vi "LockinDAQ.Trigger.vi"(8 "error in (no error)":errorcluster, 11 "LockinDAQ":refnum<class "LockinDAQ.lvclass">) -> (0 "error out":errorcluster, 3 "LockinDAQ out":refnum<class "LockinDAQ.lvclass">)   [LabVIEW 2016, in "LockinDAQ.lvclass"]
uses:
  LockinDAQ.lvclass
  Typedefs/DAQType-enum.ctl
  LockinDAQ.lvclass/LockinDAQ.ctl
  <vilib>/DAQmx/configure/trigger.llb/DAQmx Start Trigger (Digital Edge).vi
  <resource>/objmgr/daqmx.rc
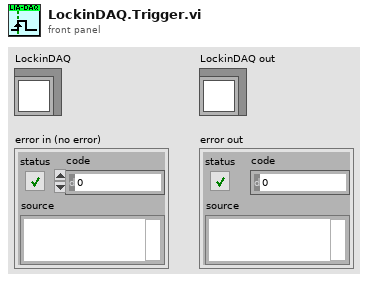
[diagram p1: front panel]
types:
  T1 = typedef "LockinDAQ.lvclass/DAQType-enum.ctl" = enum16{"None", "USB 4431", "PXI 446x"}
  T2 = cluster{"DAQ Type":T1, "master task":refnum<k21>, "RefClk.Src":tag, "SyncPulse.Src":tag, "Trigger.Src":tag, "SyncPulse.SyncTime":dbl}
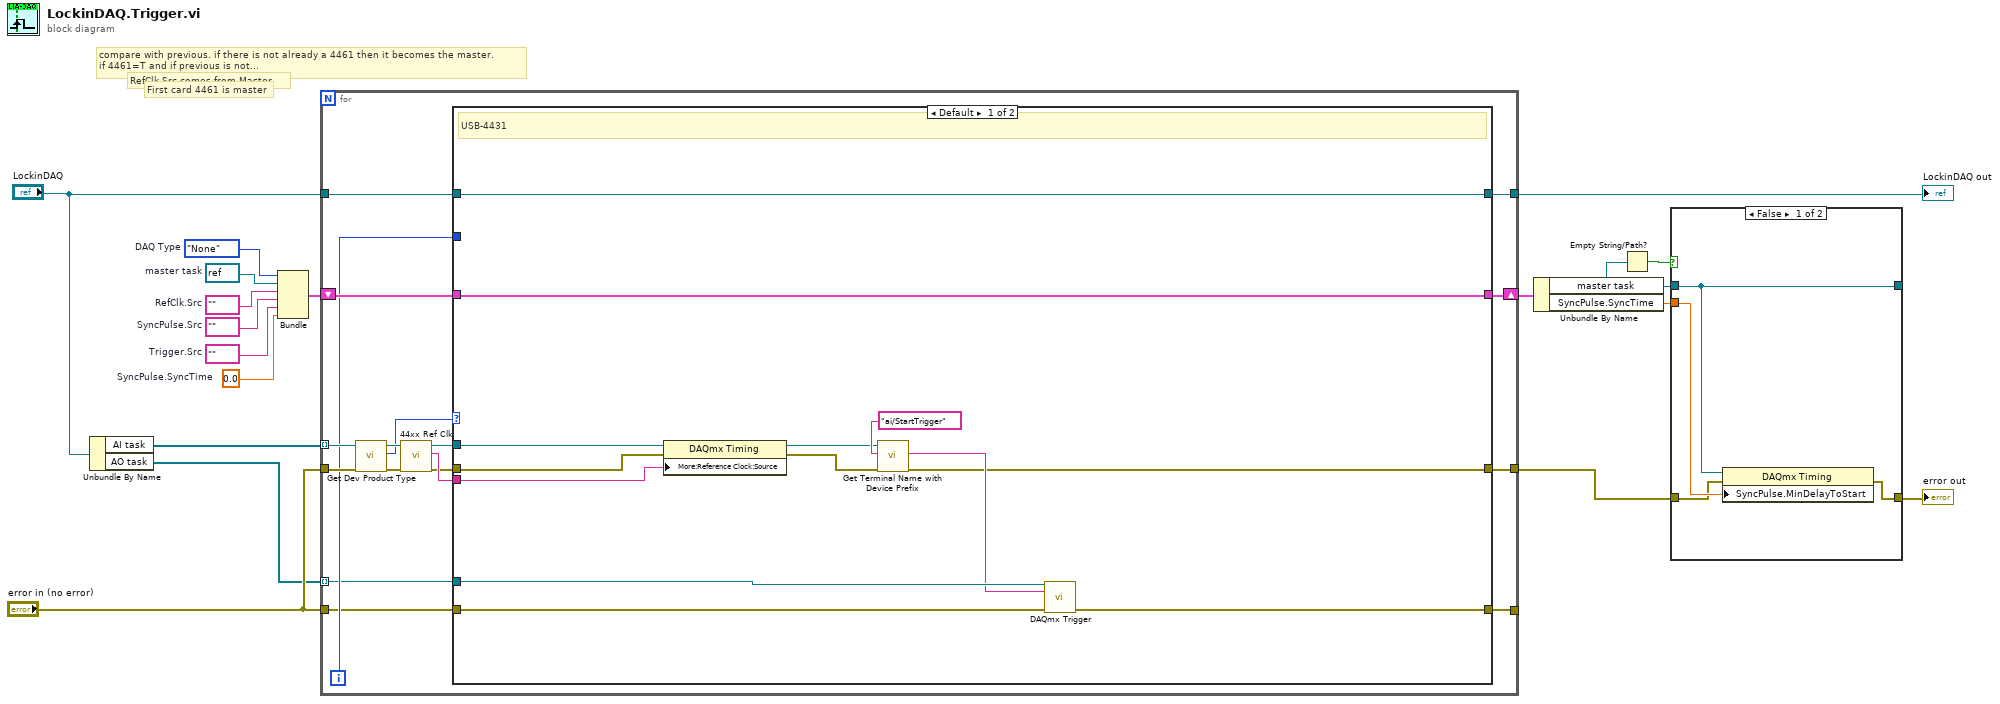
[diagram p0: block diagram]
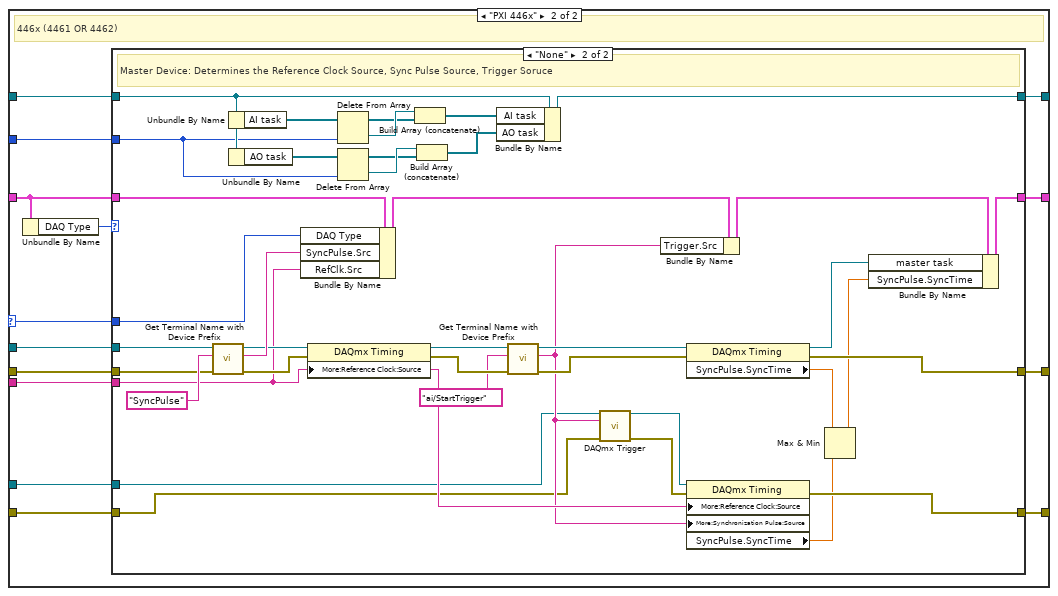
[diagram p2: hidden frame]
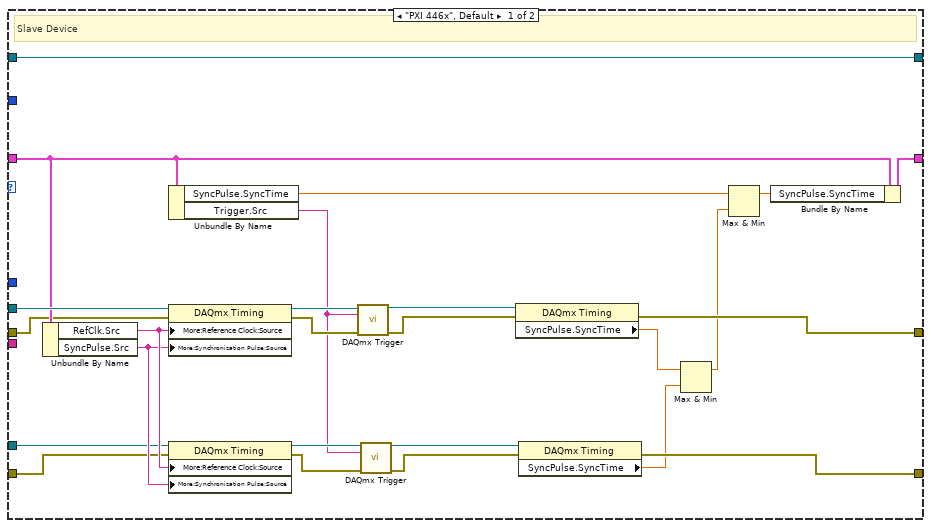
[diagram p3: hidden frame]
diagram:
  w2 = refnum<k21> refnum  # master task
  w12 = 0.0  # SyncPulse.SyncTime
  w11 = tag ""  # Trigger.Src
  w10 = tag ""  # SyncPulse.Src
  w3 = tag ""  # RefClk.Src
  w1 = DAQType-enum."None"  # DAQ Type
  # "RefClk.Src comes from Master"
  # "compare with previous. if there is not already a 4461 then it becomes the master. \nif 4461=T and if previous is not..."
  # "First card 4461 is master"
  n1 = Unbundle By Name("LockinDAQ") -> ("AI task"=w6:refnum<k21>[], "AO task"=w4:refnum<k21>[])
  n2 = Bundle("DAQ Type"=w1, "master task"=w2, "RefClk.Src"=w3, "SyncPulse.Src"=w10, "Trigger.Src"=w11, "SyncPulse.SyncTime"=w12) -> (w9:T2)  [unwired: 1 in]
  n3 = for {
    tunnel: w6 -> [w35] mode=indexing
    tunnel: "error in (no error)" -> [w32]
    shift-right: [w28] -> w13
    shift-left: w9 -> [w31]
    tunnel: [w26] -> w17
    tunnel: "LockinDAQ" -> [w25]
    tunnel: [w23] -> w7
    tunnel: [w22] -> _
    tunnel: "error in (no error)" -> [w21]
    tunnel: w4 -> [w20] mode=indexing
    i -> [w24]
    n4 = call "Get Dev Product Type.vi"("error in (no error)"=w32, "Refnum in"=w35) -> ("error out"=w34:errorcluster, "DAQ Type"=w19:T1, "Refnum out"=w33:refnum<k21>)  [unwired: 6 in, 1 out]
    n5 = call "44xx Ref Clk.vi"("error in (no error)"=w34, "Refnum in"=w33) -> ("error out"=w27:errorcluster, "RefClk.Src"=w29:tag, "Refnum out"=w30:refnum<k21>)  [unwired: 7 in]
    n6 = case shown="Default" w19 {
      selector: w19 -> [_ w59]
      tunnel: w31 -> [w48 w60]
      tunnel: w30 -> [w47 w62]
      tunnel: w29 -> [w46 w61]
      tunnel: [w48 w58] -> w28
      tunnel: w27 -> [w45 w57]
      tunnel: [w36 w56] -> w26
      tunnel: w25 -> [w44 w54]
      tunnel: w24 -> [_ w53]
      tunnel: [w44 w52] -> w23
      tunnel: [w37 w49] -> w22
      tunnel: w21 -> [w38 w51]
      tunnel: w20 -> [w40 w50]
      frame Default {
        # "USB-4431"
        n7 = property class="DAQmx Timing"(reference=w47, error in=w45, "More:Reference Clock:Source"=w46) -> (reference out=w42:refnum<k21>, error out=w41:errorcluster)
        n8 = call "Get Terminal Name with Device Prefix.vi"("error in (no error)"=w41, "Local Terminal Name"="ai/StartTrigger", "task/channels in"=w42) -> ("error out"=w36:errorcluster, "Terminal Name with Device Prefix"=w39:tag)  [unwired: 6 in, 1 out]
        n9 = call-poly <vilib>:"DAQmx Trigger.vi"("task/channels in"=w40, "source"=w39, "error in"=w38) -> ("error out"=w37:errorcluster)  [unwired: 11 in, 1 out]
      }
      frame "PXI 446x" {
        # "446x (4461 OR 4462)"
        n10 = Unbundle By Name(w60) -> ("DAQ Type"=w55:T1)
        n11 = case shown="\"None\"" w55 {
          tunnel: w62 -> [w87 w126]
          tunnel: w61 -> [_ w103]
          tunnel: w60 -> [w84 w125]
          tunnel: w59 -> [_ w124]
          tunnel: [w83 w113] -> w58
          tunnel: w57 -> [w70 w121]
          tunnel: [w81 w112] -> w56
          tunnel: w54 -> [w80 w101]
          tunnel: w53 -> [_ w100]
          tunnel: [w80 w104] -> w52
          tunnel: w51 -> [w69 w90]
          tunnel: w50 -> [w77 w91]
          tunnel: [w68 w102] -> w49
          frame "PXI 446x", Default {
            # "Slave Device"
            n12 = Unbundle By Name(w84) -> ("RefClk.Src"=w79:tag, "SyncPulse.Src"=w78:tag)
            n13 = Unbundle By Name(w84) -> ("SyncPulse.SyncTime"=w65:dbl, "Trigger.Src"=w73:tag)
            n14 = property class="DAQmx Timing"(reference=w87, error in=w70, "More:Reference Clock:Source"=w79, "More:Synchronization Pulse:Source"=w78) -> (reference out=w86:refnum<k21>, error out=w74:errorcluster)
            n15 = property class="DAQmx Timing"(reference=w77, error in=w69, "More:Reference Clock:Source"=w79, "More:Synchronization Pulse:Source"=w78) -> (reference out=w75:refnum<k21>, error out=w72:errorcluster)
            n16 = call-poly <vilib>:"DAQmx Trigger.vi"("task/channels in"=w86, "source"=w73, "error in"=w74) -> ("task out"=w85:refnum<k21>, "error out"=w82:errorcluster)  [unwired: 11 in]
            n17 = call-poly <vilib>:"DAQmx Trigger.vi"("task/channels in"=w75, "source"=w73, "error in"=w72) -> ("task out"=w76:refnum<k21>, "error out"=w71:errorcluster)  [unwired: 11 in]
            n18 = property class="DAQmx Timing"(reference=w85, error in=w82) -> (error out=w81:errorcluster, "SyncPulse.SyncTime"=w63:dbl)  [unwired: 1 out]
            n19 = property class="DAQmx Timing"(reference=w76, error in=w71) -> (error out=w68:errorcluster, "SyncPulse.SyncTime"=w67:dbl)  [unwired: 1 out]
            n20 = Max & Min(x=w63, y=w67) -> (max(x,y)=w66:dbl)  [unwired: 1 out]
            n21 = Max & Min(x=w65, y=w66) -> (max(x,y)=w64:dbl)  [unwired: 1 out]
            n22 = Bundle By Name(cluster=w84, "SyncPulse.SyncTime"=w64) -> (w83:T2)
          }
          frame "None" {
            # "Master Device: Determines the Reference Clock Source, Sync Pulse Source, Trigger Soruce"
            n23 = call "Get Terminal Name with Device Prefix.vi"("error in (no error)"=w121, "Local Terminal Name"="SyncPulse", "task/channels in"=w126) -> ("error out"=w120:errorcluster, "Terminal Name with Device Prefix"=w122:tag, "task out"=w110:refnum<k21>)  [unwired: 6 in]
            n24 = Unbundle By Name(w101) -> ("AI task"=w108:refnum<k21>[])
            n25 = Unbundle By Name(w101) -> ("AO task"=w99:refnum<k21>[])
            n26 = Bundle By Name(cluster=w125, "DAQ Type"=w124, "SyncPulse.Src"=w122, "RefClk.Src"=w103) -> (w116:T2)
            n27 = property class="DAQmx Timing"(reference=w110, error in=w120, "More:Reference Clock:Source"=w103) -> (reference out=w117:refnum<k21>, error out=w119:errorcluster)
            n28 = Delete From Array(array=w108, index=w100) -> (deleted portion=w107:refnum<k21>, array with subset deleted=w106:refnum<k21>[])  [unwired: 1 in]
            n29 = Delete From Array(array=w99, index=w100) -> (deleted portion=w98:refnum<k21>, array with subset deleted=w97:refnum<k21>[])  [unwired: 1 in]
            n30 = Build Array (concatenate)(w107, w106) -> (w105:refnum<k21>[])
            n31 = Build Array (concatenate)(w98, w97) -> (w96:refnum<k21>[])
            n32 = Bundle By Name(cluster=w101, "AI task"=w105, "AO task"=w96) -> (w104:refnum<class "LockinDAQ.lvclass">)
            n33 = call "Get Terminal Name with Device Prefix.vi"("error in (no error)"=w119, "Local Terminal Name"="ai/StartTrigger", "task/channels in"=w117) -> ("error out"=w114:errorcluster, "Terminal Name with Device Prefix"=w92:tag, "task out"=w115:refnum<k21>)  [unwired: 6 in]
            n34 = call-poly <vilib>:"DAQmx Trigger.vi"("task/channels in"=w91, "source"=w92, "error in"=w90) -> ("task out"=w88:refnum<k21>, "error out"=w89:errorcluster)  [unwired: 11 in]
            n35 = Bundle By Name(cluster=w116, "Trigger.Src"=w92) -> (w111:T2)
            n36 = property class="DAQmx Timing"(reference=w115, error in=w114) -> (reference out=w109:refnum<k21>, error out=w112:errorcluster, "SyncPulse.SyncTime"=w95:dbl)
            n37 = property class="DAQmx Timing"(reference=w88, error in=w89, "More:Reference Clock:Source"=w103, "More:Synchronization Pulse:Source"=w92) -> (error out=w102:errorcluster, "SyncPulse.SyncTime"=w94:dbl)  [unwired: 1 out]
            n38 = Max & Min(x=w95, y=w94) -> (max(x,y)=w93:dbl)  [unwired: 1 out]
            n39 = Bundle By Name(cluster=w111, "master task"=w109, "SyncPulse.SyncTime"=w93) -> (w113:T2)
          }
        }
      }
    }
  }
  "LockinDAQ out" <- w7
  n40 = Unbundle By Name(w13) -> ("master task"=w15:refnum<k21>, "SyncPulse.SyncTime"=w16:dbl)
  n41 = Empty String/Path?(string/path=w15) -> (empty?=w14:bool)
  n42 = case shown="False" w14 {
    tunnel: w15 -> [w127 w131]
    tunnel: w16 -> [w130 _]
    tunnel: w17 -> [w129 w132]
    tunnel: [w128 w132] -> w18
    tunnel: [w127 w131] -> _
    frame False {
      n43 = property class="DAQmx Timing"(reference=w127, error in=w129, "SyncPulse.MinDelayToStart"=w130) -> (error out=w128:errorcluster)  [unwired: 1 out]
    }
    frame True {
      # "If master task=empty, then no master devices were ever found (ie, all 4431s)"
    }
  }
  "error out" <- w18
